vi "UdatePortsCluster.vi"(1 "Numeric 2":i8, 2 "Input Names":string[](array[string]), 3 "Ports Array":cluster{"String":string, "Array 2":bool[]}[](array[cluster]), 4 "index":i32) -> (0 "INP Ports Array 2":cluster{"String":string, "Array 2":bool[]}[](array[cluster]))   [LabVIEW 2019]
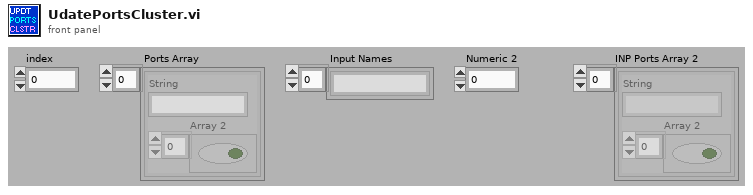
[diagram p1: front panel]
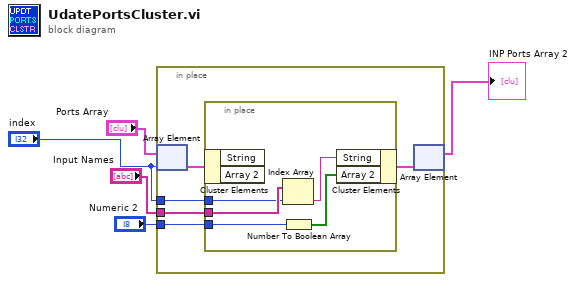
[diagram p0: block diagram]
diagram:
  n1 = in-place {
    in-place-border: "Input Names" -> [w9]
    in-place-border: "Numeric 2" -> [w8]
    in-place-border: "index" -> [w7]
    n2 = in-place-array #1("Ports Array", "index") -> (w10:cluster{"String":string, "Array 2":bool[]})
    n3 = in-place {
      in-place-border: w9 -> [w13]
      in-place-border: w8 -> [w15]
      in-place-border: w7 -> [w12]
      n4 = in-place-cluster #2(w10) -> ()  [unwired: 2 out]
      n5 = Index Array(array=w13, index=w12) -> (element=w11:string)
      n6 = Number To Boolean Array(number=w15) -> (Boolean array=w14:bool[])
      n7 = in-place-cluster #2("String"=w11, "Array 2"=w14) -> (w6:cluster{"String":string, "Array 2":bool[]})
    }
    n8 = in-place-array #1(w6) -> (→"INP Ports Array 2":cluster{"String":string, "Array 2":bool[]}[])  [unwired: 1 out]
  }
